vi "ItemsToContent.vi"(8 "error in (no error)":errorcluster, 9 "Items":refnum<class "ILabVIEWItem.lvclass">[](array[class]), 11 "CGrapherDGML in":refnum<class "CGrapherDGML.lvclass">) -> (0 "error out":errorcluster, 1 "Export string":string, 3 "CGrapherDGML out":refnum<class "CGrapherDGML.lvclass">)   [LabVIEW 2020, in "DefaultExtensions.lvlib" / "CGrapherDGML.lvclass"]
uses:
  CGrapherDGML.lvclass
  LabVIEWObjectInterfaces/ILabVIEWItem/ILabVIEWItem.lvclass
  LabVIEWObjectInterfaces/IDependencyItemRule/IDependencyItemRule.lvclass
  b016bb59-2839-43ba-88ac-4ccb6dd19c69.vi
  9977de17-27be-4ed4-afc7-a70dd966d660.vi
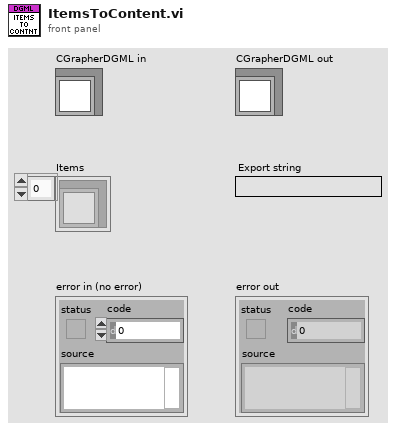
[diagram p1: front panel]
types:
  T1 = typedef "LabVIEWItem.lvlib/CLabVIEWItem.lvclass/ConnectionSet.ctl" = set{string}
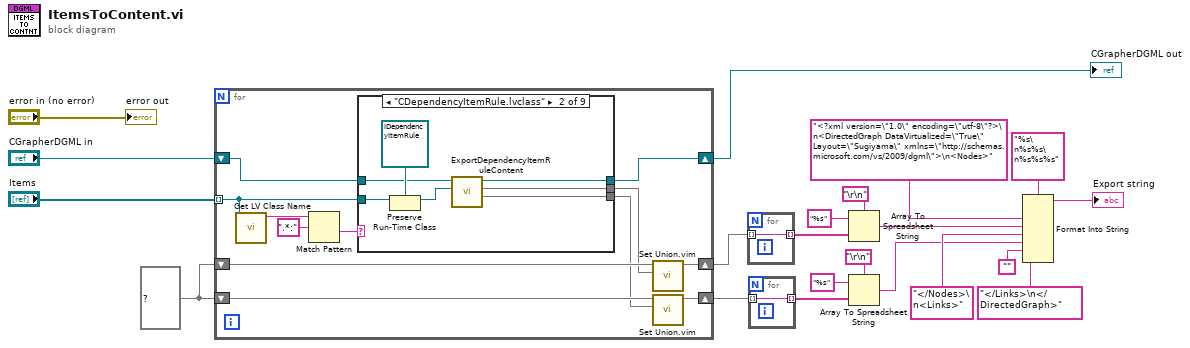
[diagram p0: block diagram]
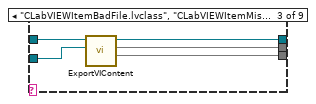
[diagram p3: hidden frame]
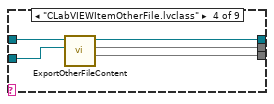
[diagram p4: hidden frame]
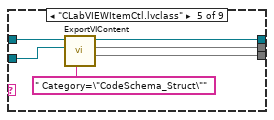
[diagram p5: hidden frame]
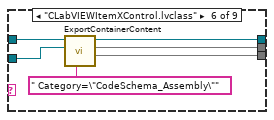
[diagram p6: hidden frame]
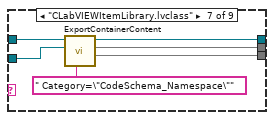
[diagram p7: hidden frame]
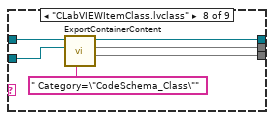
[diagram p8: hidden frame]
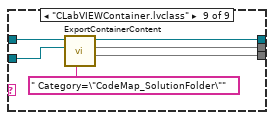
[diagram p9: hidden frame]
diagram:
  w5 = set{string} {} ("union")
  n1 = for {
    tunnel: "Items" -> [w22] mode=indexing
    shift-right: [w29] -> w3
    shift-left: w5 -> [w30]
    shift-right: [w27] -> w4
    shift-left: w5 -> [w28]
    shift-right: [w23] -> w1
    shift-left: "CGrapherDGML in" -> [w24]
    n2 = call <vilib>:"Get LV Class Name.vi"("object"=w22) -> ("class name"=w33:string)  [unwired: 9 in, 1 out]
    n3 = Match Pattern(string=w33, regular expression=".*:") -> (after substring=w31:string)  [unwired: 1 in, 3 out]
    n4 = case shown="\"CDependencyItemRule.lvclass\"" w31 {
      tunnel: w22 -> [_ w41 w44 w48 w54 w59 w65 w72 w77]
      tunnel: [_ w39 w46 w51 w53 w63 w69 w75 w81] -> w26
      tunnel: [_ w38 w45 w50 w52 w62 w68 w74 w80] -> w25
      tunnel: w24 -> [w34 w36 w43 w49 w56 w60 w66 w71 w78]
      tunnel: [w34 w35 w42 w47 w55 w58 w64 w70 w76] -> w23
      frame Default {
      }
      frame "CDependencyItemRule.lvclass" {
        n5 = Preserve Run-Time Class(object in=w41, 2:refnum<class "IDependencyItemRule.lvclass"> refnum ("IDependencyItemRule in")) -> (object out=w37:refnum<class "IDependencyItemRule.lvclass">)  [unwired: 1 in, 1 out]
        n6 = call-dynamic "ExportDependencyItemRuleContent.vi"("IDependencyItemRule in"=w37, "CGrapherDGML in"=w36) -> ("Links"=w38:T1, "Nodes"=w39:T1, "CGrapherDGML"=w35:refnum<class "CGrapherDGML.lvclass">)  [unwired: 6 in, 1 out]
      }
      frame "CLabVIEWItemBadFile.lvclass", "CLabVIEWItemMissingFile.lvclass", "CLabVIEWItemVI.lvclass", "CLabVIEWItemVIM.lvclass" {
        n7 = call-dynamic "ExportVIContent.vi"("ILabVIEWItem in"=w44, "CGrapherDGML in"=w43) -> ("Links"=w45:T1, "Nodes"=w46:T1, "CGrapherDGML"=w42:refnum<class "CGrapherDGML.lvclass">)  [unwired: 7 in]
      }
      frame "CLabVIEWItemOtherFile.lvclass" {
        n8 = call-dynamic "ExportOtherFileContent.vi"("ILabVIEWItem in"=w48, "CGrapherDGML in"=w49) -> ("Links"=w50:T1, "Nodes"=w51:T1, "CGrapherDGML"=w47:refnum<class "CGrapherDGML.lvclass">)  [unwired: 6 in, 1 out]
      }
      frame "CLabVIEWItemCtl.lvclass" {
        n9 = call-dynamic "ExportVIContent.vi"("CodeSchema"=" Category=\"CodeSchema_Struct\"", "ILabVIEWItem in"=w54, "CGrapherDGML in"=w56) -> ("Links"=w52:T1, "Nodes"=w53:T1, "CGrapherDGML"=w55:refnum<class "CGrapherDGML.lvclass">)  [unwired: 6 in]
      }
      frame "CLabVIEWItemXControl.lvclass" {
        n10 = call-dynamic "ExportContainerContent.vi"("CodeSchema"=" Category=\"CodeSchema_Assembly\"", "ILabVIEWItem in"=w59, "CGrapherDGML in"=w60) -> ("Links"=w62:T1, "Nodes"=w63:T1, "CGrapherDGML"=w58:refnum<class "CGrapherDGML.lvclass">)  [unwired: 5 in, 1 out]
      }
      frame "CLabVIEWItemLibrary.lvclass" {
        n11 = call-dynamic "ExportContainerContent.vi"("CodeSchema"=" Category=\"CodeSchema_Namespace\"", "ILabVIEWItem in"=w65, "CGrapherDGML in"=w66) -> ("Links"=w68:T1, "Nodes"=w69:T1, "CGrapherDGML"=w64:refnum<class "CGrapherDGML.lvclass">)  [unwired: 5 in, 1 out]
      }
      frame "CLabVIEWItemClass.lvclass" {
        n12 = call-dynamic "ExportContainerContent.vi"("CodeSchema"=" Category=\"CodeSchema_Class\"", "ILabVIEWItem in"=w72, "CGrapherDGML in"=w71) -> ("Links"=w74:T1, "Nodes"=w75:T1, "CGrapherDGML"=w70:refnum<class "CGrapherDGML.lvclass">)  [unwired: 5 in, 1 out]
      }
      frame "CLabVIEWContainer.lvclass" {
        n13 = call-dynamic "ExportContainerContent.vi"("CodeSchema"=" Category=\"CodeMap_SolutionFolder\"", "ILabVIEWItem in"=w77, "CGrapherDGML in"=w78) -> ("Links"=w80:T1, "Nodes"=w81:T1, "CGrapherDGML"=w76:refnum<class "CGrapherDGML.lvclass">)  [unwired: 5 in, 1 out]
      }
    }
    n14 = call "Set Union.vim"("set 2"=w26, "set 1"=w30) -> ("union"=w29:set{string})  [unwired: 9 in]
    n15 = call "Set Union.vim"("set 2"=w25, "set 1"=w28) -> ("union"=w27:set{string})  [unwired: 9 in]
  }
  "CGrapherDGML out" <- w1
  n16 = for {
    tunnel: [w82] -> w7 mode=indexing
    tunnel: w3 -> [w82] mode=indexing
  }
  n17 = for {
    tunnel: [w83] -> w6 mode=indexing
    tunnel: w4 -> [w83] mode=indexing
  }
  n18 = Array To Spreadsheet String(delimiter (Tab)="\r\n", array=w7, 3:"%s" ("format string")) -> (spreadsheet string=w12:string)
  n19 = Array To Spreadsheet String(delimiter (Tab)="\r\n", array=w6, 3:"%s" ("format string")) -> (spreadsheet string=w9:string)
  n20 = Format Into String(format string="%s\n%s%s\n%s%s%s", "<?xml version=\"1.0\" encoding=\"utf-8\"?>\n<DirectedGraph DataVirtualized=\"True\" Layout=\"Sugiyama\" xmlns=\"http://schemas.microsoft.com/vs/2009/dgml\">\n<Nodes>", w12, "</Nodes>\n<Links>" ("format string"), w9, "", "</Links>\n</DirectedGraph>") -> (resulting string=→"Export string":string)  [unwired: 2 in, 1 out]
  "error out" <- "error in (no error)"
